vi "Facade.vi"(0 "Data In":T5, 2 "Display State In":T3, 3 "Container State":T4) -> (6 "Data Out":T5, 7 "Display State Out":T3, 8 "Action":T2)   [LabVIEW 2019, in "XAOMsetting.xctl"]
uses:
  XAOMsetting.xctl
  Data.ctl
  <vilib>/_xctls/Container State.ctl
  State.ctl
  <vilib>/_xctls/Action.ctl
  <vilib>/_xctls/XControlSupport.lvlib
panel:
  in  "AOMsetting":T1
  # "Manual :"
  # "Automatic :"
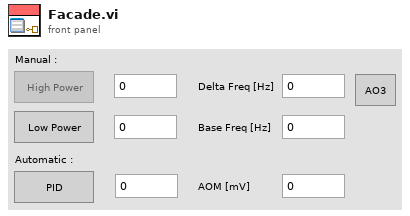
[diagram p1: front panel]
types:
  T1 = cluster{"HighPower":bool, "LowPower":bool, "PID":bool, "HighPowerNum":dbl, "LowPowerNum":dbl, "PIDnum":dbl, "DeltaFreq":dbl, "BaseFreq":dbl, "AOMout":dbl, "AO3":bool}
  T2 = typedef "XControlSupport.lvlib/Action.ctl" = cluster{"Data Changed?":bool, "State Changed?":bool, "Action Name":string}
  T3 = typedef "XAOMsetting.xctl/State.ctl" = cluster{"ButtonSelected":enum16{"PID", "Low", "High"}}
  T4 = typedef "XControlSupport.lvlib/Container State.ctl" = cluster{"Indicator?":bool, "Run Mode?":bool, " Refnum":refnum<vi>}
  T5 = typedef "XAOMsetting.xctl/Data.ctl" = cluster{"HighPowerNum":dbl, "LowPowerNum":dbl, "PIDnum":dbl, "DeltaFreq":dbl, "BaseFreq":dbl, "AOMout":dbl, "ButtonSelected":enum16{"PID", "Low", "High"}, "AO3":bool}
  T6 = enum8{"Enabled", "Disabled", "Disabled and Grayed Out"}
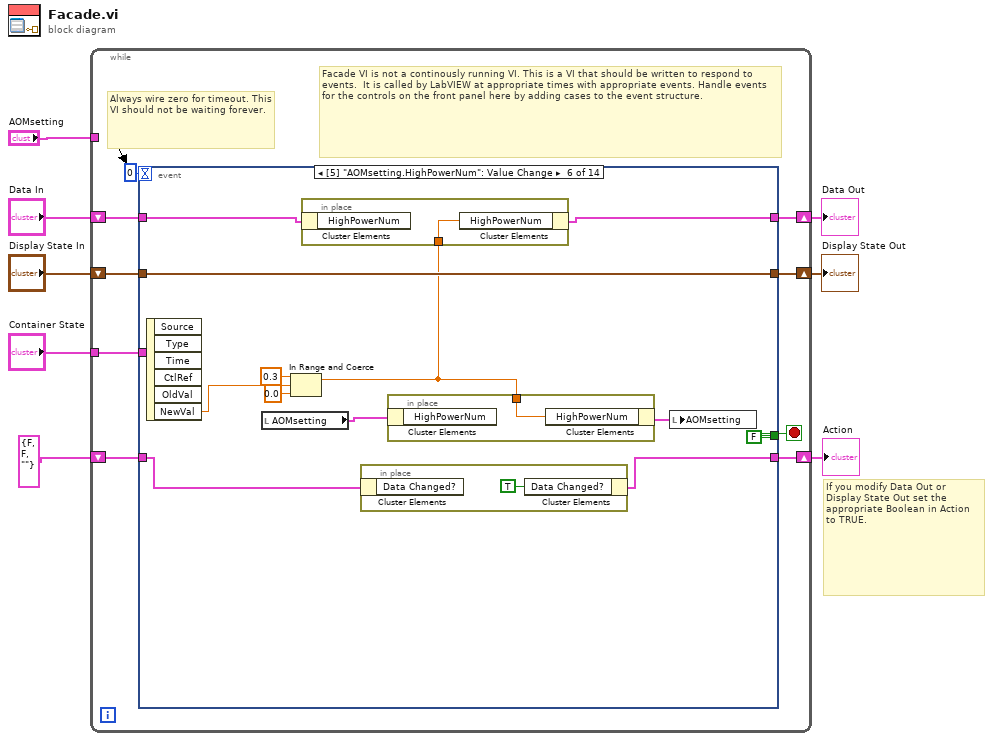
[diagram p0: block diagram]
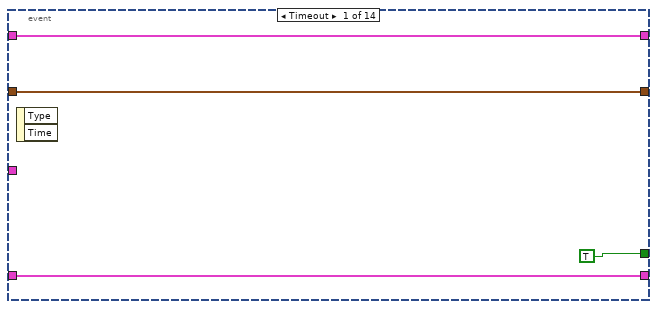
[diagram p2: hidden frame]
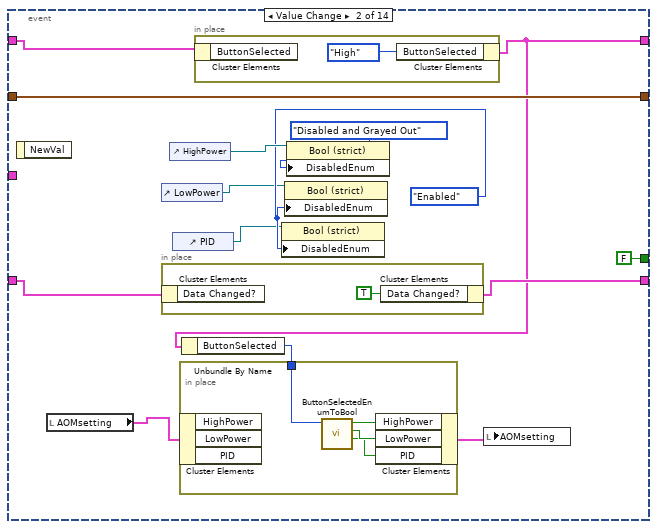
[diagram p3: hidden frame]
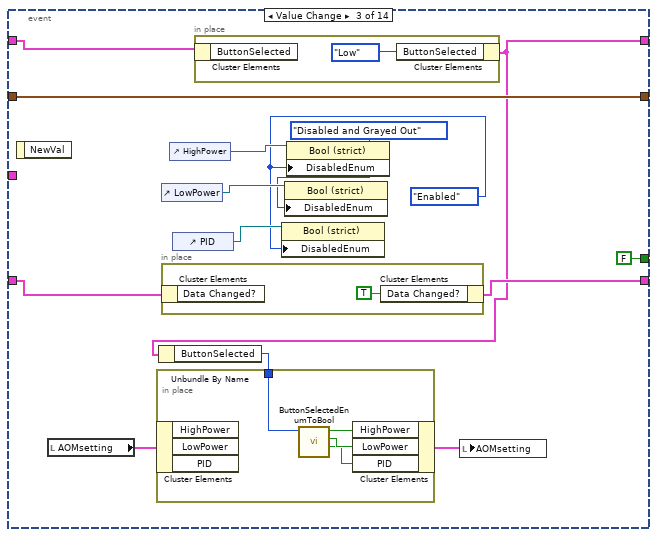
[diagram p4: hidden frame]
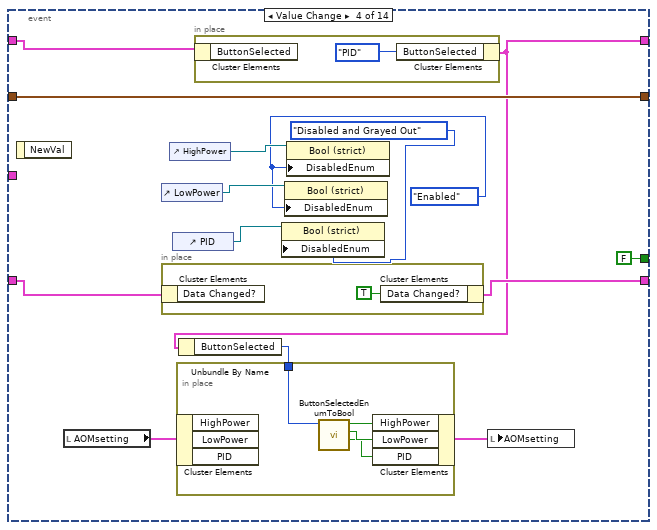
[diagram p5: hidden frame]
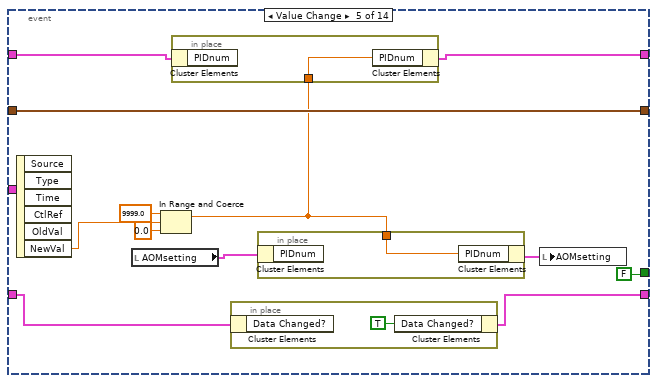
[diagram p6: hidden frame]
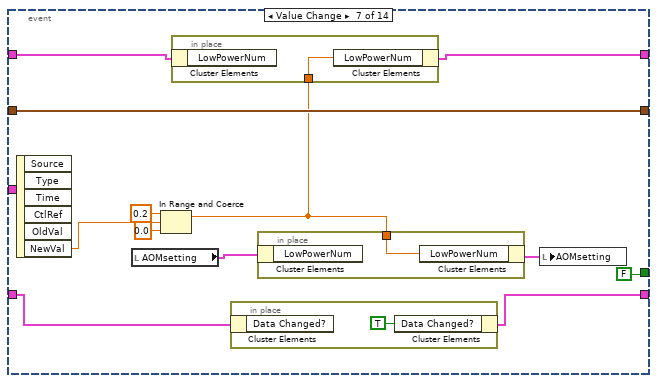
[diagram p7: hidden frame]
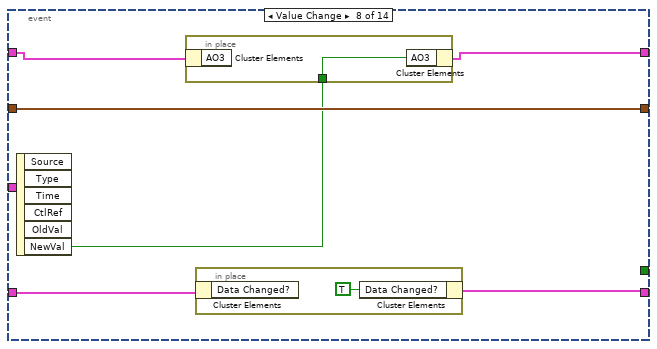
[diagram p8: hidden frame]
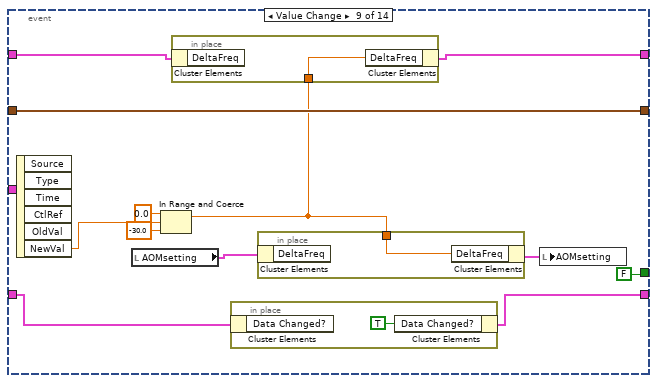
[diagram p9: hidden frame]
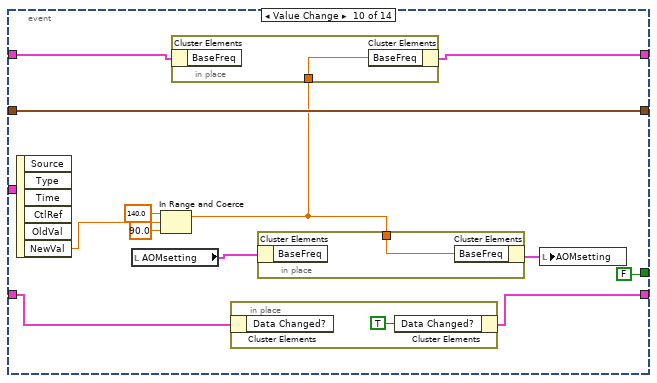
[diagram p10: hidden frame]
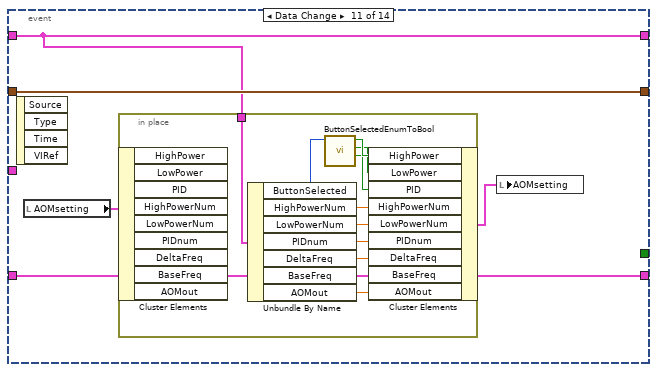
[diagram p11: hidden frame]
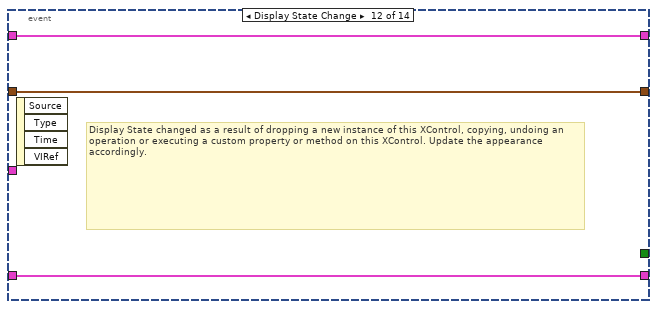
[diagram p12: hidden frame]
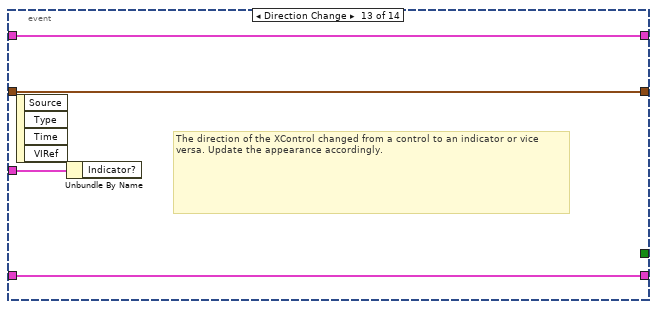
[diagram p13: hidden frame]
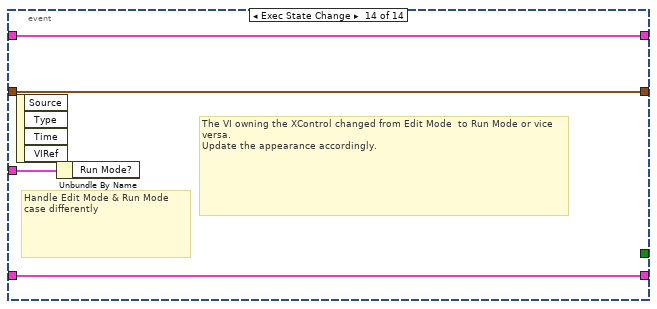
[diagram p14: hidden frame]
diagram:
  # "If you modify Data Out or\nDisplay State Out set the\nappropriate Boolean in Action\nto TRUE."
  n1 = while {
    shift-right: [w16] -> w5
    shift-left: "Display State In" -> [w17]
    tunnel: "Container State" -> [w13]
    shift-right: [w12] -> w8
    shift-left: "Data In" -> [w9]
    shift-right: [w10] -> w3
    shift-left: T2 {"Data Changed?"=FALSE, "State Changed?"=FALSE, "Action Name"=""} ("Action") -> [w11]
    tunnel: "AOMsetting" -> [_]
    stop <- w15 stop-if-true
    # "Facade VI is not a continously running VI. This is a VI that should be written to respond to events.  It is called by LabVIEW at appropriate times with appropriate events. Handle events for the controls on the front panel here by adding cases to the event structure."
    # "Always wire zero for timeout. This\nVI should not be waiting forever."
    n2 = event shown="[5] \"AOMsetting.HighPowerNum\": Value Change" {
      selector: _ -> [_ _ _ _ _ _ _ _ _ _ _ _ _ _]
      dyn-events: _ -> [_ _ _ _ _ _ _ _ _ _ _ _ _ _]
      timeout: 0 -> [_ _ _ _ _ _ _ _ _ _ _ _ _ _]
      tunnel: w17 -> [w19 w35 w55 w75 w93 w108 w123 w132 w146 w161 w169 w183 w186 w190]
      tunnel: [w19 w35 w55 w75 w93 w108 w123 w132 w146 w161 w169 w183 w186 w190] -> w16
      tunnel: [TRUE FALSE FALSE FALSE FALSE FALSE FALSE _ FALSE FALSE _ _ _ _] -> w15
      tunnel: w13 -> [_ _ _ _ _ _ _ _ _ _ _ _ w187 w191]
      tunnel: w9 -> [w18 w29 w51 w71 w88 w103 w118 w131 w141 w156 w165 w182 w185 w189]
      tunnel: [w18 w22 w44 w64 w86 w101 w116 w130 w139 w154 w165 w182 w185 w189] -> w12
      tunnel: [w20 w27 w49 w69 w82 w97 w112 w127 w135 w150 w168 w181 w184 w188] -> w10
      tunnel: w11 -> [w20 w28 w50 w70 w83 w98 w113 w128 w136 w151 w168 w181 w184 w188]
      event Timeout {
        n3 = event-data() -> ()  [unwired: 1 in, 2 out]
      }
      event "AOMsetting.HighPower": Value Change {
        w32 = T6."Enabled" ("Disabled")
        n4 = event-data() -> ()  [unwired: 1 in, 1 out]
        n5 = local read "AOMsetting"() -> (w23:T1)
        n6 = control-ref of="LowPower"() -> (w30:refnum<vi>)
        n7 = in-place {
          n8 = in-place-cluster #1(w28) -> ()  [unwired: 1 out]
          n9 = in-place-cluster #1("Data Changed?"=TRUE) -> (w27:T2)
        }
        n10 = control-ref of="HighPower"() -> (w34:refnum<vi>)
        n11 = control-ref of="PID"() -> (w31:refnum<vi>)
        n12 = in-place {
          n13 = in-place-cluster #2(w29) -> ()  [unwired: 1 out]
          n14 = in-place-cluster #2("ButtonSelected"=enum16{"PID", "Low", "High"}."High") -> (w22:T5)
        }
        n15 = Unbundle By Name(w22) -> ("ButtonSelected"=w25:enum16{"PID", "Low", "High"})
        n16 = in-place {
          in-place-border: w25 -> [w39]
          n17 = in-place-cluster #3(w23) -> ()  [unwired: 3 out]
          n18 = call "ButtonSelectedEnumToBool.vi"("ButtonSelected"=w39) -> ("PID"=w36:bool, "Low"=w37:bool, "High"=w38:bool)  [unwired: 8 in]
          n19 = in-place-cluster #3("HighPower"=w38, "LowPower"=w37, "PID"=w36) -> (w24:T1)
        }
        n20 = property class="Bool (strict)"(reference=w31, "DisabledEnum"=w32) -> ()  [unwired: 1 in, 2 out]
        n21 = property class="Bool (strict)"(reference=w30, "DisabledEnum"=w32) -> ()  [unwired: 1 in, 2 out]
        n22 = property class="Bool (strict)"(reference=w34, "DisabledEnum"=T6."Disabled and Grayed Out" ("Disabled")) -> ()  [unwired: 1 in, 2 out]
        n23 = local write "AOMsetting"(w24) -> ()
      }
      event "AOMsetting.LowPower": Value Change {
        w46 = T6."Enabled" ("Disabled")
        n24 = event-data() -> ()  [unwired: 1 in, 1 out]
        n25 = local read "AOMsetting"() -> (w43:T1)
        n26 = control-ref of="LowPower"() -> (w52:refnum<vi>)
        n27 = in-place {
          n28 = in-place-cluster #4(w50) -> ()  [unwired: 1 out]
          n29 = in-place-cluster #4("Data Changed?"=TRUE) -> (w49:T2)
        }
        n30 = control-ref of="HighPower"() -> (w54:refnum<vi>)
        n31 = control-ref of="PID"() -> (w53:refnum<vi>)
        n32 = in-place {
          n33 = in-place-cluster #5(w51) -> ()  [unwired: 1 out]
          n34 = in-place-cluster #5("ButtonSelected"=enum16{"PID", "Low", "High"}."Low") -> (w44:T5)
        }
        n35 = Unbundle By Name(w44) -> ("ButtonSelected"=w45:enum16{"PID", "Low", "High"})
        n36 = in-place {
          in-place-border: w45 -> [w59]
          n37 = in-place-cluster #6(w43) -> ()  [unwired: 3 out]
          n38 = call "ButtonSelectedEnumToBool.vi"("ButtonSelected"=w59) -> ("PID"=w56:bool, "Low"=w57:bool, "High"=w58:bool)  [unwired: 8 in]
          n39 = in-place-cluster #6("HighPower"=w58, "LowPower"=w57, "PID"=w56) -> (w42:T1)
        }
        n40 = property class="Bool (strict)"(reference=w53, "DisabledEnum"=w46) -> ()  [unwired: 1 in, 2 out]
        n41 = property class="Bool (strict)"(reference=w52, "DisabledEnum"=T6."Disabled and Grayed Out" ("Disabled")) -> ()  [unwired: 1 in, 2 out]
        n42 = property class="Bool (strict)"(reference=w54, "DisabledEnum"=w46) -> ()  [unwired: 1 in, 2 out]
        n43 = local write "AOMsetting"(w42) -> ()
      }
      event "AOMsetting.PID": Value Change {
        w67 = T6."Enabled" ("Disabled")
        n44 = event-data() -> ()  [unwired: 1 in, 1 out]
        n45 = local read "AOMsetting"() -> (w63:T1)
        n46 = control-ref of="LowPower"() -> (w72:refnum<vi>)
        n47 = in-place {
          n48 = in-place-cluster #7(w70) -> ()  [unwired: 1 out]
          n49 = in-place-cluster #7("Data Changed?"=TRUE) -> (w69:T2)
        }
        n50 = control-ref of="HighPower"() -> (w74:refnum<vi>)
        n51 = control-ref of="PID"() -> (w73:refnum<vi>)
        n52 = in-place {
          n53 = in-place-cluster #8(w71) -> ()  [unwired: 1 out]
          n54 = in-place-cluster #8("ButtonSelected"=enum16{"PID", "Low", "High"}."PID") -> (w64:T5)
        }
        n55 = Unbundle By Name(w64) -> ("ButtonSelected"=w65:enum16{"PID", "Low", "High"})
        n56 = in-place {
          in-place-border: w65 -> [w79]
          n57 = in-place-cluster #9(w63) -> ()  [unwired: 3 out]
          n58 = call "ButtonSelectedEnumToBool.vi"("ButtonSelected"=w79) -> ("PID"=w76:bool, "Low"=w77:bool, "High"=w78:bool)  [unwired: 8 in]
          n59 = in-place-cluster #9("HighPower"=w78, "LowPower"=w77, "PID"=w76) -> (w62:T1)
        }
        n60 = property class="Bool (strict)"(reference=w73, "DisabledEnum"=T6."Disabled and Grayed Out" ("Disabled")) -> ()  [unwired: 1 in, 2 out]
        n61 = property class="Bool (strict)"(reference=w72, "DisabledEnum"=w67) -> ()  [unwired: 1 in, 2 out]
        n62 = property class="Bool (strict)"(reference=w74, "DisabledEnum"=w67) -> ()  [unwired: 1 in, 2 out]
        n63 = local write "AOMsetting"(w62) -> ()
      }
      event "AOMsetting.PIDnum": Value Change {
        n64 = event-data() -> ("NewVal"=w92:dbl)  [unwired: 1 in, 5 out]
        n65 = local read "AOMsetting"() -> (w89:T1)
        n66 = In Range and Coerce(upper limit=9999.0, x=w92, lower limit=0.0) -> (coerced(x)=w87:dbl)  [unwired: 1 out]
        n67 = in-place {
          in-place-border: w87 -> [w95]
          n68 = in-place-cluster #10(w88) -> ()  [unwired: 1 out]
          n69 = in-place-cluster #10("PIDnum"=w95) -> (w86:T5)
        }
        n70 = in-place {
          n71 = in-place-cluster #11(w83) -> ()  [unwired: 1 out]
          n72 = in-place-cluster #11("Data Changed?"=TRUE) -> (w82:T2)
        }
        n73 = in-place {
          in-place-border: w87 -> [w96]
          n74 = in-place-cluster #12(w89) -> ()  [unwired: 1 out]
          n75 = in-place-cluster #12("PIDnum"=w96) -> (w85:T1)
        }
        n76 = local write "AOMsetting"(w85) -> ()
      }
      event "AOMsetting.HighPowerNum": Value Change {
        n77 = event-data() -> ("NewVal"=w107:dbl)  [unwired: 1 in, 5 out]
        n78 = local read "AOMsetting"() -> (w104:T1)
        n79 = In Range and Coerce(upper limit=0.3, x=w107, lower limit=0.0) -> (coerced(x)=w102:dbl)  [unwired: 1 out]
        n80 = in-place {
          in-place-border: w102 -> [w110]
          n81 = in-place-cluster #13(w103) -> ()  [unwired: 1 out]
          n82 = in-place-cluster #13("HighPowerNum"=w110) -> (w101:T5)
        }
        n83 = in-place {
          n84 = in-place-cluster #14(w98) -> ()  [unwired: 1 out]
          n85 = in-place-cluster #14("Data Changed?"=TRUE) -> (w97:T2)
        }
        n86 = in-place {
          in-place-border: w102 -> [w111]
          n87 = in-place-cluster #15(w104) -> ()  [unwired: 1 out]
          n88 = in-place-cluster #15("HighPowerNum"=w111) -> (w100:T1)
        }
        n89 = local write "AOMsetting"(w100) -> ()
      }
      event "AOMsetting.LowPowerNum": Value Change {
        n90 = event-data() -> ("NewVal"=w122:dbl)  [unwired: 1 in, 5 out]
        n91 = local read "AOMsetting"() -> (w119:T1)
        n92 = In Range and Coerce(upper limit=0.2, x=w122, lower limit=0.0) -> (coerced(x)=w117:dbl)  [unwired: 1 out]
        n93 = in-place {
          in-place-border: w117 -> [w125]
          n94 = in-place-cluster #16(w118) -> ()  [unwired: 1 out]
          n95 = in-place-cluster #16("LowPowerNum"=w125) -> (w116:T5)
        }
        n96 = in-place {
          n97 = in-place-cluster #17(w113) -> ()  [unwired: 1 out]
          n98 = in-place-cluster #17("Data Changed?"=TRUE) -> (w112:T2)
        }
        n99 = in-place {
          in-place-border: w117 -> [w126]
          n100 = in-place-cluster #18(w119) -> ()  [unwired: 1 out]
          n101 = in-place-cluster #18("LowPowerNum"=w126) -> (w115:T1)
        }
        n102 = local write "AOMsetting"(w115) -> ()
      }
      event "AOMsetting.AO3": Value Change {
        n103 = event-data() -> ("NewVal"=w129:bool)  [unwired: 1 in, 5 out]
        n104 = in-place {
          in-place-border: w129 -> [w134]
          n105 = in-place-cluster #19(w131) -> ()  [unwired: 1 out]
          n106 = in-place-cluster #19("AO3"=w134) -> (w130:T5)
        }
        n107 = in-place {
          n108 = in-place-cluster #20(w128) -> ()  [unwired: 1 out]
          n109 = in-place-cluster #20("Data Changed?"=TRUE) -> (w127:T2)
        }
      }
      event "AOMsetting.DeltaFreq": Value Change {
        n110 = event-data() -> ("NewVal"=w145:dbl)  [unwired: 1 in, 5 out]
        n111 = local read "AOMsetting"() -> (w142:T1)
        n112 = In Range and Coerce(upper limit=0.0, x=w145, lower limit=-30.0) -> (coerced(x)=w140:dbl)  [unwired: 1 out]
        n113 = in-place {
          in-place-border: w140 -> [w148]
          n114 = in-place-cluster #21(w141) -> ()  [unwired: 1 out]
          n115 = in-place-cluster #21("DeltaFreq"=w148) -> (w139:T5)
        }
        n116 = in-place {
          n117 = in-place-cluster #22(w136) -> ()  [unwired: 1 out]
          n118 = in-place-cluster #22("Data Changed?"=TRUE) -> (w135:T2)
        }
        n119 = in-place {
          in-place-border: w140 -> [w149]
          n120 = in-place-cluster #23(w142) -> ()  [unwired: 1 out]
          n121 = in-place-cluster #23("DeltaFreq"=w149) -> (w138:T1)
        }
        n122 = local write "AOMsetting"(w138) -> ()
      }
      event "AOMsetting.BaseFreq": Value Change {
        n123 = event-data() -> ("NewVal"=w160:dbl)  [unwired: 1 in, 5 out]
        n124 = local read "AOMsetting"() -> (w157:T1)
        n125 = In Range and Coerce(upper limit=140.0, x=w160, lower limit=90.0) -> (coerced(x)=w155:dbl)  [unwired: 1 out]
        n126 = in-place {
          in-place-border: w155 -> [w163]
          n127 = in-place-cluster #24(w156) -> ()  [unwired: 1 out]
          n128 = in-place-cluster #24("BaseFreq"=w163) -> (w154:T5)
        }
        n129 = in-place {
          n130 = in-place-cluster #25(w151) -> ()  [unwired: 1 out]
          n131 = in-place-cluster #25("Data Changed?"=TRUE) -> (w150:T2)
        }
        n132 = in-place {
          in-place-border: w155 -> [w164]
          n133 = in-place-cluster #26(w157) -> ()  [unwired: 1 out]
          n134 = in-place-cluster #26("BaseFreq"=w164) -> (w153:T1)
        }
        n135 = local write "AOMsetting"(w153) -> ()
      }
      event Data Change {
        n136 = event-data() -> ()  [unwired: 1 in, 4 out]
        n137 = local read "AOMsetting"() -> (w167:T1)
        n138 = in-place {
          in-place-border: w165 -> [w180]
          n139 = in-place-cluster #27(w167) -> ()  [unwired: 9 out]
          n140 = Unbundle By Name(w180) -> ("ButtonSelected"=w173:enum16{"PID", "Low", "High"}, "HighPowerNum"=w179:dbl, "LowPowerNum"=w178:dbl, "PIDnum"=w177:dbl, "DeltaFreq"=w176:dbl, "BaseFreq"=w175:dbl, "AOMout"=w174:dbl)
          n141 = call "ButtonSelectedEnumToBool.vi"("ButtonSelected"=w173) -> ("PID"=w170:bool, "Low"=w171:bool, "High"=w172:bool)  [unwired: 8 in]
          n142 = in-place-cluster #27("HighPower"=w172, "LowPower"=w171, "PID"=w170, "HighPowerNum"=w179, "LowPowerNum"=w178, "PIDnum"=w177, "DeltaFreq"=w176, "BaseFreq"=w175, "AOMout"=w174) -> (w166:T1)
        }
        n143 = local write "AOMsetting"(w166) -> ()
      }
      event Display State Change {
        # "Display State changed as a result of dropping a new instance of this XControl, copying, undoing an operation or executing a custom property or method on this XControl. Update the appearance accordingly."
        n144 = event-data() -> ()  [unwired: 1 in, 4 out]
      }
      event Direction Change {
        # "The direction of the XControl changed from a control to an indicator or vice versa. Update the appearance accordingly."
        n145 = event-data() -> ()  [unwired: 1 in, 4 out]
        n146 = Unbundle By Name(w187) -> ()  [unwired: 1 out]
      }
      event Exec State Change {
        # "The VI owning the XControl changed from Edit Mode  to Run Mode or vice versa.\nUpdate the appearance accordingly."
        # "Handle Edit Mode & Run Mode\ncase differently"
        n147 = event-data() -> ()  [unwired: 1 in, 4 out]
        n148 = Unbundle By Name(w191) -> ()  [unwired: 1 out]
      }
    }
  }
  "Display State Out" <- w5
  "Data Out" <- w8
  "Action" <- w3
